vi "single cycle simple kalman step.vi"(0 "state in":T1, 1 "apply measurement":bool, 5 "location":T4, 9 "pixel values cluster":T3, 11 "feedback channel":enum16{"channel 0", "channel 1", "both"}(ring)=enum."both") -> (4 "state out":T1)   [LabVIEW 2010]
uses:
  kalman 3-axis state.ctl
  kalman simple pv state.ctl
  common_typedefs/channels_cluster.ctl
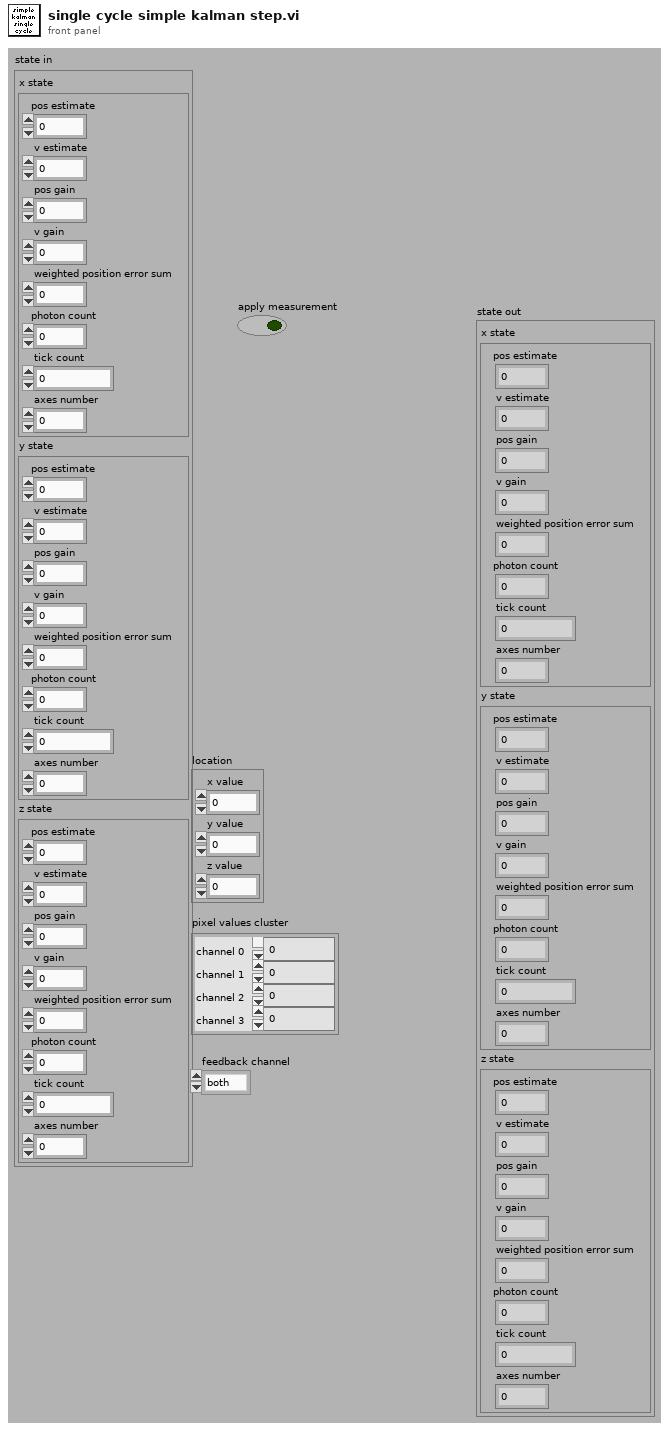
[diagram p1: front panel]
types:
  T1 = typedef "kalman 3-axis state.ctl" = cluster{"x state":T2, "y state":T2, "z state":T2}
  T2 = typedef "kalman simple pv state.ctl" = cluster{"pos estimate":fxp<+/-,32,16>, "v estimate":fxp<+/-,32,-4>, "pos gain":fxp<+,32,0>, "v gain":fxp<+,32,0>, "weighted position error sum":fxp<+/-,32,32>, "photon count":u32, "tick count":u32, "axes number":u8}
  T3 = typedef "channels_cluster.ctl" = cluster{"channel 0":u32, "channel 1":u32, "channel 2":u32, "channel 3":u32}
  T4 = cluster{"x value":i16, "y value":i16, "z value":i16}
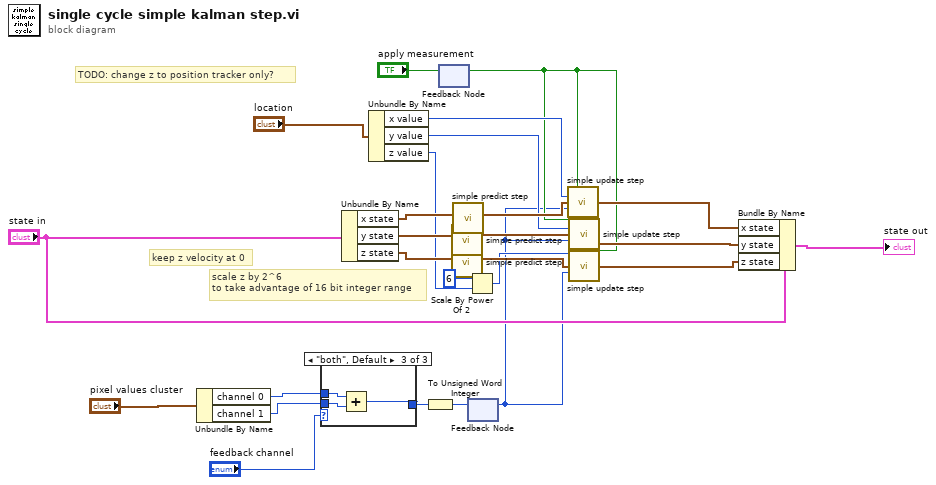
[diagram p0: block diagram]
diagram:
  # "TODO: change z to position tracker only?"
  # "keep z velocity at 0"
  # "scale z by 2^6\nto take advantage of 16 bit integer range"
  n1 = Unbundle By Name("pixel values cluster") -> ("channel 0"=w11:u32, "channel 1"=w10:u32)
  n2 = case shown="\"both\", Default" "feedback channel" {
    tunnel: w11 -> [w27 _ w31]
    tunnel: w10 -> [_ w28 w30]
    tunnel: [w27 w28 w29] -> w4
    frame "channel 0" {
    }
    frame "channel 1" {
    }
    frame "both", Default {
      n3 = Add(x=w31, y=w30) -> (x+y=w29:u32)
    }
  }
  n4 = Unbundle By Name("state in") -> ("x state"=w26:T2, "y state"=w25:T2, "z state"=w24:T2)
  n5 = Unbundle By Name("location") -> ("x value"=w23:i16, "y value"=w19:i16, "z value"=w18:i16)
  n6 = To Unsigned Word Integer(number=w4) -> (unsigned 16bit integer=w3:u16)
  n7 = feedback-in #1("apply measurement") -> ()
  n8 = feedback #1() -> (w7:bool)  [unwired: 1 in]
  n9 = call "simple predict step.vi"("state in"=w25) -> ("state out"=w21:T2)  [unwired: 10 in]
  n10 = call "simple predict step.vi"("state in"=w24) -> ("state out"=w20:T2)  [unwired: 10 in]
  n11 = call "simple predict step.vi"("state in"=w26) -> ("state out"=w22:T2)  [unwired: 10 in]
  n12 = Scale By Power Of 2(n=6, x=w18) -> (x*2^n=w16:i16)
  n13 = feedback-in #2(w3) -> ()
  n14 = feedback #2() -> (w2:u16)  [unwired: 1 in]
  n15 = call "simple update step.vi"("apply measurement?"=w7, "location"=w23, "state in"=w22, "num photons"=w2) -> ("state out"=w15:T2)  [unwired: 11 in]
  n16 = call "simple update step.vi"("apply measurement?"=w7, "location"=w19, "state in"=w21, "num photons"=w2) -> ("state out"=w14:T2)  [unwired: 11 in]
  n17 = call "simple update step.vi"("apply measurement?"=w7, "location"=w16, "state in"=w20, "num photons"=w2) -> ("state out"=w13:T2)  [unwired: 11 in]
  n18 = Bundle By Name(cluster="state in", "x state"=w15, "y state"=w14, "z state"=w13) -> (→"state out":T1)
